vi "Increment Count in Cell.vi"(0 "1D Board":T1[](array[typedef]), 5 "Cell Index":i32, 7 "Team Number":i32, 11 "error in (no error)":errorcluster) -> (4 "1D Board Out":T1[](array[typedef]), 6 "Coins Won":i32, 15 "error out":errorcluster)   [LabVIEW 2014, in "Dragon Tamers.lvlib"]
uses:
  Dragon Tamers.lvlib
  Typedefs/Board Cell.ctl
  Typedefs/Cell Occupancy.ctl
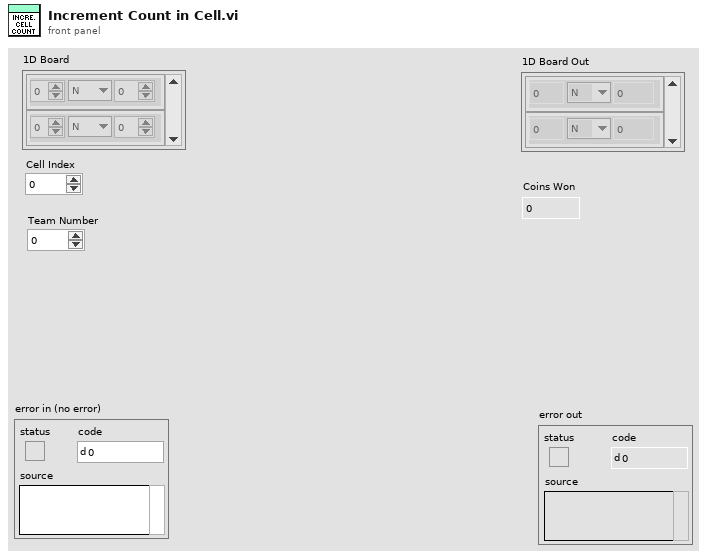
[diagram p1: front panel]
types:
  T1 = typedef "Dragon Tamers.lvlib/Board Cell.ctl" = cluster{"Team":i32, "Occu.":T2, "Count":i32}
  T2 = typedef "Dragon Tamers.lvlib/Cell Occupancy.ctl" = enum16{"N", "C", "K"}
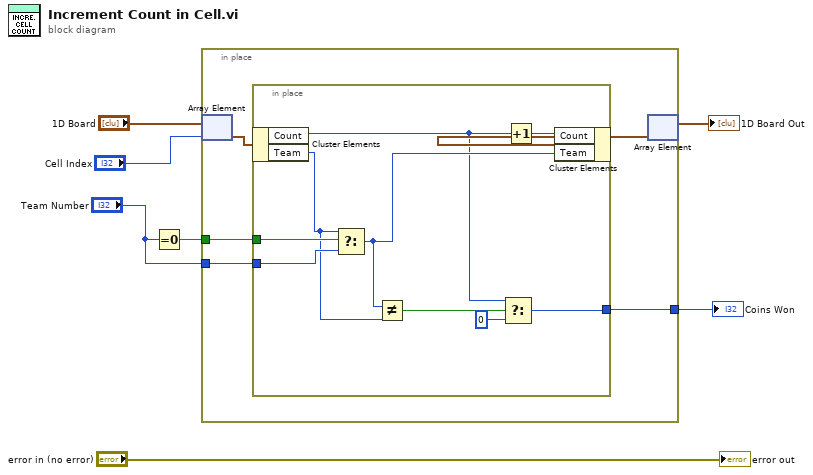
[diagram p0: block diagram]
diagram:
  n1 = Equal To 0?(x="Team Number") -> (x = 0?=w2:bool)
  n2 = in-place {
    in-place-border: "Team Number" -> [w10]
    in-place-border: w2 -> [w9]
    in-place-border: [w8] -> w1
    n3 = in-place-array #1("1D Board", "Cell Index") -> (w12:T1)
    n4 = in-place {
      in-place-border: w10 -> [w19]
      in-place-border: w9 -> [w20]
      in-place-border: [w13] -> w8
      n5 = in-place-cluster #2(w12) -> ("Count"=w16:i32, "Team"=w17:i32)
      n6 = Select(t=w17, s=w20, f=w19) -> (s? t:f=w18:i32)
      n7 = Not Equal?(x=w18, y=w17) -> (x != y?=w15:bool)
      n8 = Select(t=w16, s=w15, f=0) -> (s? t:f=w13:i32)
      n9 = Increment(x=w16) -> (x+1=w21:i32)
      n10 = in-place-cluster #2("Count"=w21, "Team"=w18) -> (w11:T1)
    }
    n11 = in-place-array #1(w11) -> (→"1D Board Out":T1[])  [unwired: 1 out]
  }
  "Coins Won" <- w1
  "error out" <- "error in (no error)"
